vi "LabVIEWDemo.vi"() -> ()   [LabVIEW 2017]
uses:
  C:/Program Files (x86)/Wasatch Photonics/Wasatch.NET/WasatchNET.dll
panel:
  out "Last Error":string
  in  "Detector Setpoint (°C)":dbl
  out "Detector TEC (°C)":dbl format="%.2f"
  out "Serial Number":string
  out "Model":string
  in  "Integration Time (ms)":u32=100 min=10 max=5000 step=1
  out "Excitation (nm)":dbl
  out "Coeff3":dbl
  out "Coeff2":dbl
  out "Coeff1":dbl
  out "Coeff0":dbl
  in  "Start/Stop":bool
  out "XY Graph":T1(graph)
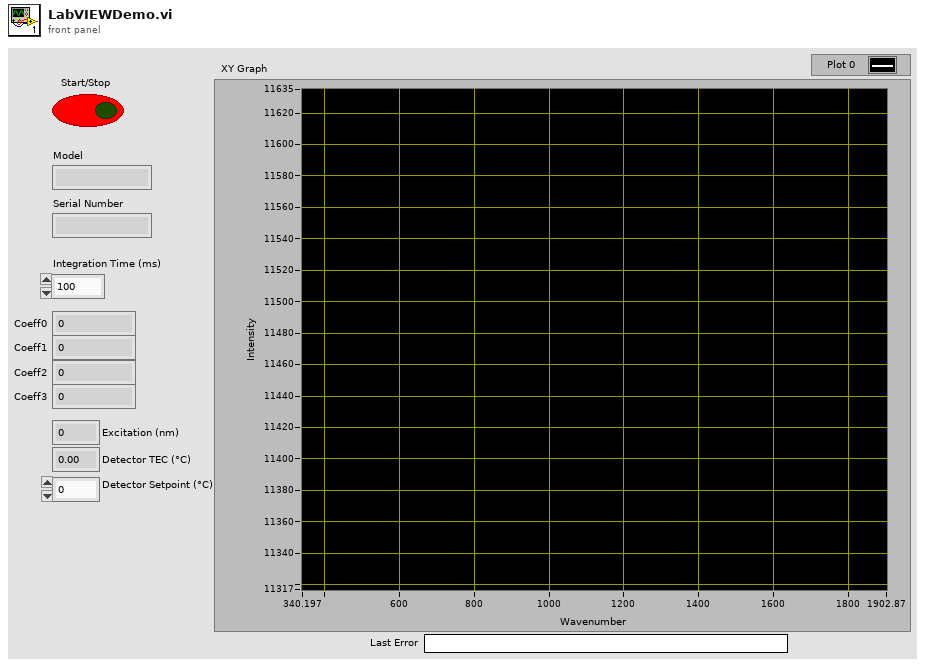
[diagram p1: front panel]
types:
  T1 = cluster{"getSpectrum":dbl[], "wavenumbers":dbl[]}
  T2 = cluster{"wavenumbers":dbl[], "getSpectrum":dbl[]}
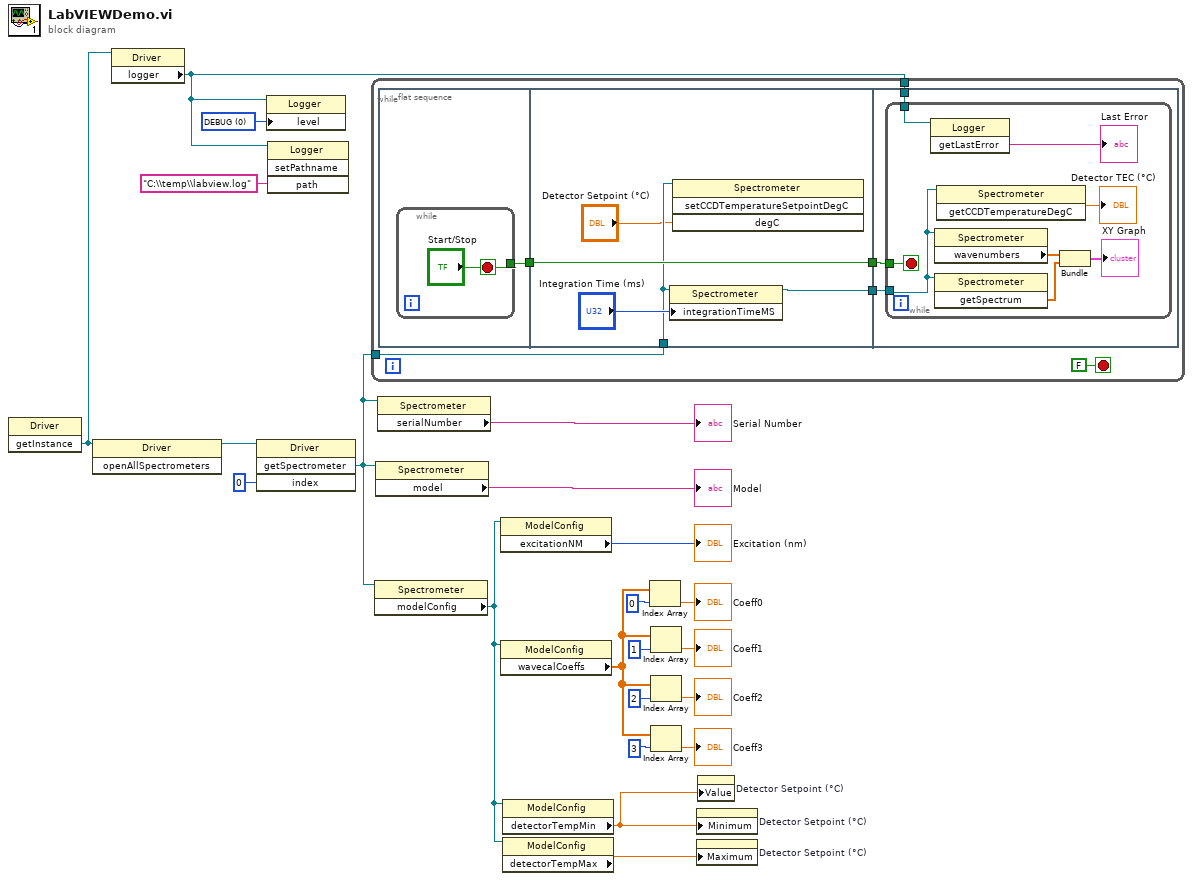
[diagram p0: block diagram]
diagram:
  w5 = 0 items=["DEBUG", "INFO", "ERROR", "NEVER"] ("level")
  n1 = invoke on="Invoke Node" class="Driver" method="getInstance"() -> ("getInstance"=w8:refnum<k24>)  [unwired: 3 in, 2 out]
  n2 = invoke class="Driver" method="openAllSpectrometers"(reference=w8) -> (reference out=w9:refnum<k24>)  [unwired: 2 in, 2 out]
  n3 = property class="Driver"(reference=w8) -> ("logger"=w6:refnum<k24>)  [unwired: 1 in, 2 out]
  n4 = invoke on="Invoke Node" class="Driver" method="getSpectrometer"(reference=w9, "index"=0) -> ("getSpectrometer"=w4:refnum<k24>)  [unwired: 2 in, 3 out]
  n5 = property class="Logger"(reference=w6, "level"=w5) -> ()  [unwired: 1 in, 2 out]
  n6 = invoke class="Logger" method="setPathname"(reference=w6, "path"="C:\\temp\\labview.log") -> ()  [unwired: 2 in, 4 out]
  n7 = while {
    tunnel: w4 -> [w25]
    tunnel: w6 -> [w23]
    stop <- FALSE stop-if-true
    n8 = flat-sequence {
      tunnel: [w29] -> w27
      tunnel: w27 -> [w35]
      tunnel: [w35] -> w26
      tunnel: w25 -> [w32]
      tunnel: [w34] -> w24
      tunnel: w26 -> [w38]
      tunnel: w24 -> [w37]
      tunnel: w23 -> [w36]
      frame #0 {
        n9 = while {
          tunnel: ["Start/Stop"] -> w29
          stop <- "Start/Stop" stop-if-true
        }
      }
      frame #1 {
        n10 = property class="Spectrometer"(reference=w32, "integrationTimeMS"="Integration Time (ms)") -> (reference out=w34:refnum<k24>)  [unwired: 1 in, 1 out]
        n11 = invoke class="Spectrometer" method="setCCDTemperatureSetpointDegC"(reference=w32, "degC"="Detector Setpoint (°C)") -> ()  [unwired: 2 in, 4 out]
      }
      frame #2 {
        n12 = while {
          tunnel: w38 -> [w46]
          tunnel: w37 -> [w42]
          tunnel: w36 -> [w40]
          stop <- w46 stop-if-true
          n13 = invoke class="Logger" method="getLastError"(reference=w40) -> ("getLastError"=→"Last Error":string)  [unwired: 2 in, 2 out]
          n14 = property class="Spectrometer"(reference=w42) -> ("wavenumbers"=w45:dbl[])  [unwired: 1 in, 2 out]
          n15 = invoke class="Spectrometer" method="getSpectrum"(reference=w42) -> ("getSpectrum"=w44:dbl[])  [unwired: 2 in, 2 out]
          n16 = invoke class="Spectrometer" method="getCCDTemperatureDegC"(reference=w42) -> ("getCCDTemperatureDegC"=→"Detector TEC (°C)":sgl)  [unwired: 2 in, 2 out]
          n17 = Bundle("wavenumbers"=w45, "getSpectrum"=w44) -> (→"XY Graph":T2)  [unwired: 1 in]
        }
      }
    }
  }
  n18 = property class="Spectrometer"(reference=w4) -> ("modelConfig"=w2:refnum<k24>)  [unwired: 1 in, 2 out]
  n19 = property class="Spectrometer"(reference=w4) -> ("model"=→"Model":string)  [unwired: 1 in, 2 out]
  n20 = property class="Spectrometer"(reference=w4) -> ("serialNumber"=→"Serial Number":string)  [unwired: 1 in, 2 out]
  n21 = property class="ModelConfig"(reference=w2) -> ("excitationNM"=→"Excitation (nm)":i16)  [unwired: 1 in, 2 out]
  n22 = property class="ModelConfig"(reference=w2) -> ("wavecalCoeffs"=w16:sgl[])  [unwired: 1 in, 2 out]
  n23 = property class="ModelConfig"(reference=w2) -> ("detectorTempMin"=w1:sgl)  [unwired: 1 in, 2 out]
  n24 = property class="ModelConfig"(reference=w2) -> ("detectorTempMax"=w3:sgl)  [unwired: 1 in, 2 out]
  n25 = Index Array(array=w16, index=0) -> (element=→"Coeff0":sgl)
  n26 = Index Array(array=w16, index=1 ("1")) -> (element=→"Coeff1":sgl)
  n27 = Index Array(array=w16, index=2) -> (element=→"Coeff2":sgl)
  n28 = Index Array(array=w16, index=3) -> (element=→"Coeff3":sgl)
  n29 = property on="Detector Setpoint (°C)" class="DigNum (strict)"("Minimum"=w1) -> ()  [unwired: 2 in, 2 out]
  n30 = property on="Detector Setpoint (°C)" class="DigNum (strict)"("Maximum"=w3) -> ()  [unwired: 2 in, 2 out]
  n31 = property on="Detector Setpoint (°C)" class="DigNum (strict)"("Value"=w1) -> ()  [unwired: 2 in, 2 out]
